vi "VPA QC Digital Scale DAQ.vi"(8 "error in (no error)":errorcluster, 9 "Function":enum16{"Change Com Settings", "Read"}(ring), 10 "DAQ Ref Cluster":T1) -> (0 "error out":errorcluster, 2 "DAQ Ref Cluster Out":T1)   [LabVIEW 2013]
uses:
  Controls/VPA QC DAQ Ref Cluster.ctl
  Controls/VPA QC Scale Communication Settings DVR.ctl
  Controls/VPA QC Scale Communication Settings.ctl
  <vilib>/Instr/_visa.llb/VISA Configure Serial Port (Instr).vi
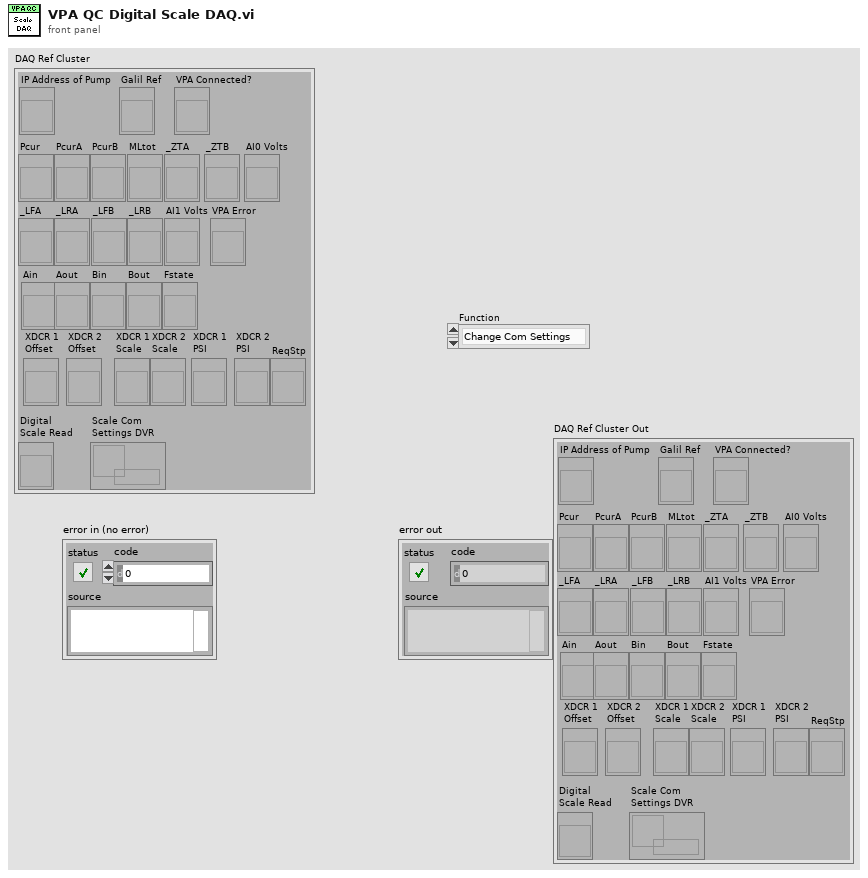
[diagram p1: front panel]
types:
  T1 = typedef "VPA QC DAQ Ref Cluster.ctl" = cluster{"IP Address of Pump":refnum<vi>, "Galil Ref":refnum<vi>, "VPA Connected?":refnum<vi>, "Pcur":refnum<vi>, "PcurA":refnum<vi>, "PcurB":refnum<vi>, "MLtot":refnum<vi>, "_LFA":refnum<vi>, "_LRA":refnum<vi>, "_LFB":refnum<vi>, "_LRB":refnum<vi>, "_ZTA":refnum<vi>, "_ZTB":refnum<vi>, "AI0 Volts":refnum<vi>, "AI1 Volts":refnum<vi>, "VPA Error":refnum<vi>, "Ain":refnum<vi>, "Aout":refnum<vi>, "Bin":refnum<vi>, "Bout":refnum<vi>, "Fstate":refnum<vi>, "XDCR 1\nOffset":refnum<vi>, "XDCR 2 \nOffset":refnum<vi>, "XDCR 1\nScale":refnum<vi>, "XDCR 2\nScale":refnum<vi>, "XDCR 1\nPSI":refnum<vi>, "XDCR 2\nPSI":refnum<vi>, "ReqStp":refnum<vi>, "Digital \nScale Read":refnum<vi>, "Scale Com\nSettings DVR":T2}
  T2 = typedef "VPA QC Scale Communication Settings DVR.ctl" = refnum<data-value>
  T3 = typedef "VPA QC Scale Communication Settings.ctl" = cluster{"Baud":i32, "Data Bits":i32, "Stop Bits":i32, "Parity":enum16{"None", "Odd", "Even", "Mark", "Space"}, "Flow Control":enum16{"None", "XON/XOFF", "RTS/CTS", "XON/XOFF & RTS/CTS", "DTR/DSR", "XON/XOFF & DTR/DSR"}, "VISA resource name":refnum<visa-resource-name>}
  T4 = enum16{"None", "XON/XOFF", "RTS/CTS", "XON/XOFF & RTS/CTS", "DTR/DSR", "XON/XOFF & DTR/DSR"}
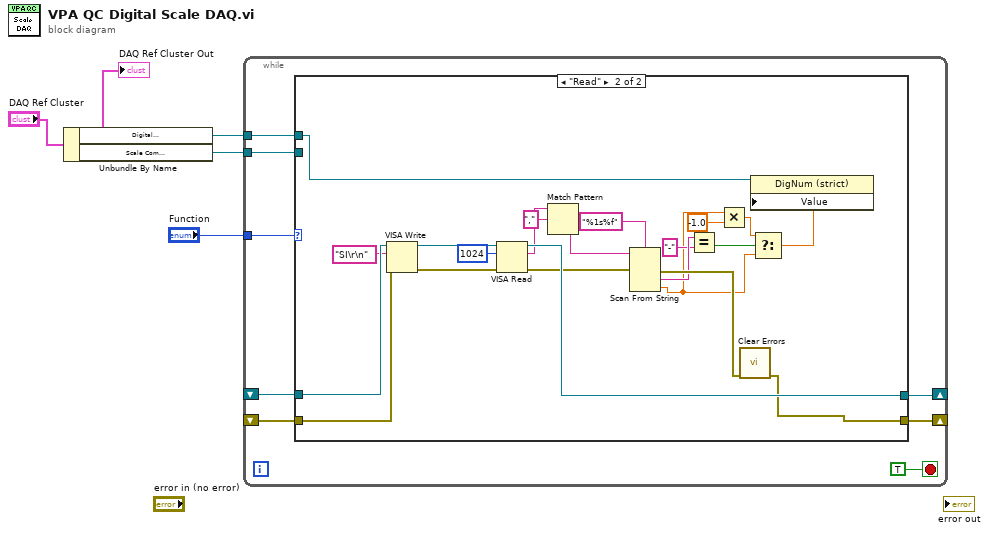
[diagram p0: block diagram]
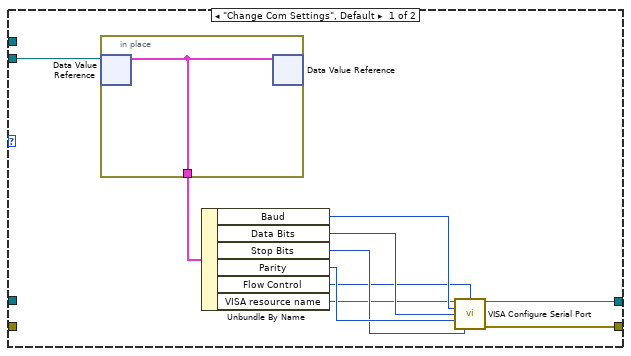
[diagram p2: hidden frame]
diagram:
  n1 = Unbundle By Name("DAQ Ref Cluster") -> ("Digital \nScale Read"=w2:refnum<vi>, "Scale Com\nSettings DVR"=w1:T2)
  n2 = while {
    tunnel: "Function" -> [w12]
    tunnel: w2 -> [w11]
    tunnel: w1 -> [w10]
    shift-right: [w8] -> _
    shift-left: _ -> [w6]
    shift-right: [w7] -> _
    shift-left: _ -> [w5]
    stop <- TRUE stop-if-true
    n3 = case shown="\"Read\"" w12 {
      tunnel: w11 -> [_ w36]
      tunnel: w10 -> [w22 _]
      tunnel: [w14 w42] -> w8
      tunnel: [w13 w37] -> w7
      tunnel: w6 -> [_ w45]
      tunnel: w5 -> [_ w41]
      frame "Change Com Settings", Default {
        n4 = in-place {
          in-place-border: [w23] -> w21
          n5 = in-place-dvr #1(w22) -> (w23:T3)  [unwired: 1 out]
          n6 = in-place-dvr #1(w23) -> ()  [unwired: 2 out]
        }
        n7 = Unbundle By Name(w21) -> ("Baud"=w20:i32, "Data Bits"=w19:i32, "Stop Bits"=w17:i32, "Parity"=w18:enum16{"None", "Odd", "Even", "Mark", "Space"}, "Flow Control"=w16:T4, "VISA resource name"=w15:refnum<visa-resource-name>)
        n8 = call-poly "VISA Configure Serial Port"("VISA resource name"=w15, "baud rate (9600)"=w20, "data bits (8)"=w19, "parity (0:none)"=w18, "stop bits (10: 1 bit)"=w17, "flow control (0:none)"=w16) -> ("VISA resource name out"=w14:refnum<visa-resource-name>, "error out"=w13:errorcluster)  [unwired: 8 in]
      }
      frame "Read" {
        n9 = VISA Write(VISA resource name=w45, write buffer="SI\r\n", error in (no error)=w41) -> (VISA resource name out=w43:refnum<visa-resource-name>, error out=w38:errorcluster)  [unwired: 1 out]
        n10 = VISA Read(VISA resource name=w43, byte count=u32 1024, error in (no error)=w38) -> (VISA resource name out=w42:refnum<visa-resource-name>, read buffer=w25:string, error out=w27:errorcluster)  [unwired: 1 out]
        n11 = Match Pattern(string=w25, regular expression=",") -> (after substring=w26:string)  [unwired: 1 in, 3 out]
        n12 = Scan From String(format string="%1s%f", input string=w26, error in=w27) -> (error out=w35:errorcluster, output 1=w34:string, output 2=w29:dbl)  [unwired: 3 in, 2 out]
        n13 = Equal?(x=w34, y="-") -> (x = y?=w30:bool)
        n14 = Multiply(x=w29, y=-1.0) -> (x*y=w31:dbl)
        n15 = call <vilib>:"Clear Errors.vi"("error in (no error)"=w35) -> ("error out"=w37:errorcluster)  [unwired: 6 in]
        n16 = Select(t=w31, s=w30, f=w29) -> (s? t:f=w28:dbl)
        n17 = property class="DigNum (strict)"(reference=w36, "Value"=w28) -> ()  [unwired: 1 in, 2 out]
      }
    }
  }
  "DAQ Ref Cluster Out" <- "DAQ Ref Cluster"
